vi "Toggle.vi"(1 "Trigger":bool) -> (0 "New Mode":bool)   [LabVIEW 2018]
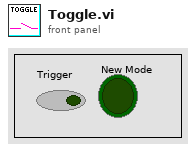
[diagram p1: front panel]
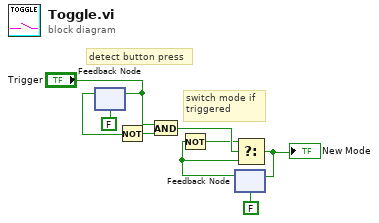
[diagram p0: block diagram]
diagram:
  # "detect button press"
  # "switch mode if\ntriggered"
  n1 = feedback-in #1("Trigger") -> ()
  n2 = feedback #1(FALSE ("Button")) -> (w5:bool)
  n3 = Not(x=w5) -> (.not. x?=w7:bool)
  n4 = And(x="Trigger", y=w7) -> (x .and. y?=w9:bool)
  n5 = feedback #2(FALSE) -> (w3:bool)
  n6 = Not(x=w3) -> (.not. x?=w8:bool)
  n7 = Select(t=w8, s=w9, f=w3) -> (s? t:f=w4:bool)
  "New Mode" <- w4
  n8 = feedback-in #2(w4) -> ()
